vi "SET_BodyText.vi"(8 "error in (no error)":errorcluster, 10 "Body Text":T1={"Line 1 text"="", "Line 2 text"="", "Line 3 text"="", "Line 4 text"="", "Line 1 color"=0, "Line 2 color"=0, "Line 3 color"=0, "Line 4 color"=0, "Body Text Spec"={"Font"="", "Alignment"=0, "Size"=3}, "Center text vertically"=FALSE, "Capitalize Text"=FALSE} {"Body Text Spec"."Alignment" items=["left", "center", "right"]}, 11 "Icon Framework.lvclass in":refnum<class "Icon Framework.lvclass">) -> (0 "error out":errorcluster, 3 "Icon Framework.lvclass out":refnum<class "Icon Framework.lvclass">)   [LabVIEW 2020, in "Icon Framework.lvclass"]
doc: "Specifies the Body Text."
uses:
  <vilib>/LabVIEW Icon API/lv_icon/Classes/Icon Framework/Icon Framework.lvclass
  <vilib>/LabVIEW Icon API/lv_icon/Controls/BodyText.ctl
  <vilib>/LabVIEW Icon API/lv_icon/Controls/Font.ctl
  <vilib>/LabVIEW Icon API/lv_icon/Controls/Alignment.ctl
  <vilib>/LabVIEW Icon API/lv_icon/Classes/Icon Framework/Icon Framework.lvclass/Icon Framework.ctl
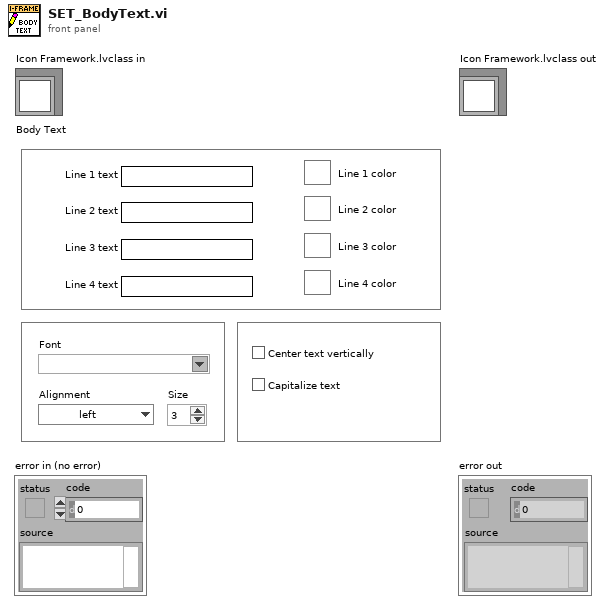
[diagram p1: front panel]
types:
  T1 = typedef "BodyText.ctl" = cluster{"Line 1 text":string, "Line 2 text":string, "Line 3 text":string, "Line 4 text":string, "Line 1 color":u32, "Line 2 color":u32, "Line 3 color":u32, "Line 4 color":u32, "Body Text Spec":cluster{"Font":T2, "Alignment":T3, "Size":u8}, "Center text vertically":bool, "Capitalize Text":bool}
  T2 = typedef "Font.ctl" = string
  T3 = typedef "Alignment.ctl" = u16
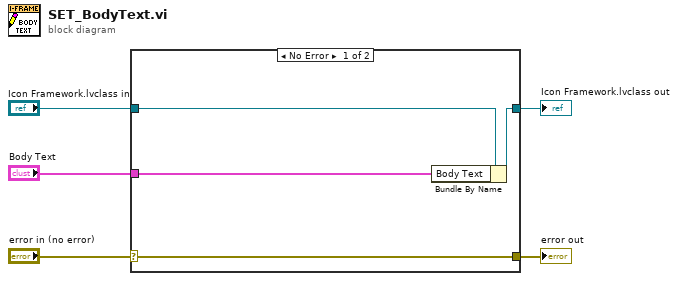
[diagram p0: block diagram]
diagram:
  n1 = case shown="No Error" "error in (no error)" {
    selector: "error in (no error)" -> [w9 w10]
    tunnel: [w9 w10] -> w4
    tunnel: [w7 w11] -> w2
    tunnel: "Icon Framework.lvclass in" -> [w8 w11]
    tunnel: "Body Text" -> [w6 _]
    frame No Error {
      n2 = Bundle By Name(cluster=w8, "Body Text"=w6) -> (w7:refnum<class "Icon Framework.lvclass">)
    }
    frame Error {
    }
  }
  "error out" <- w4
  "Icon Framework.lvclass out" <- w2
